vi "encodeByteArray.vi"(3 "ByteArray":u8[](array[numeric]) format="%.0x") -> (1 "MessagePack":u8[](array[numeric]) format="%.0x")   [LabVIEW 2015]
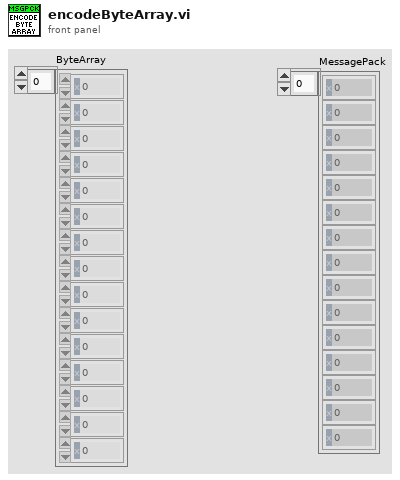
[diagram p1: front panel]
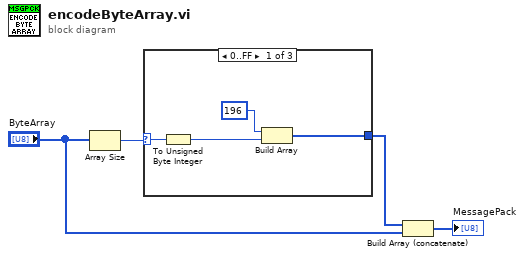
[diagram p0: block diagram]
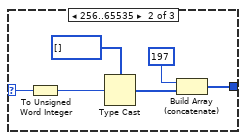
[diagram p2: hidden frame]
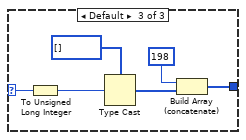
[diagram p3: hidden frame]
diagram:
  n1 = Array Size(array="ByteArray") -> (size(s)=w2:i32)
  n2 = case shown="0..FF" w2 {
    selector: w2 -> [w6 w12 w18]
    tunnel: [w7 w13 w19] -> w3
    frame 0..255 {
      n3 = To Unsigned Byte Integer(number=w6) -> (unsigned 8bit integer=w5:u8)
      n4 = Build Array(u8 196, w5) -> (w7:u8[])
    }
    frame 256..65535 {
      n5 = To Unsigned Word Integer(number=w12) -> (unsigned 16bit integer=w11:u16)
      n6 = Type Cast(type=u8[] [] ("appended array"), x=w11) -> (*(type *) &x=w9:u8[])
      n7 = Build Array (concatenate)(u8 197, w9) -> (w13:u8[])
    }
    frame Default {
      n8 = To Unsigned Long Integer(number=w18) -> (unsigned 32bit integer=w17:u32)
      n9 = Type Cast(type=u8[] [] ("appended array"), x=w17) -> (*(type *) &x=w15:u8[])
      n10 = Build Array (concatenate)(u8 198, w15) -> (w19:u8[])
    }
  }
  n11 = Build Array (concatenate)(w3, "ByteArray") -> (→"MessagePack":u8[])
